vi "Delete.vi"(8 "error in (no error)":errorcluster, 11 "ByRefClass in":refnum<class "ClassByRef.lvclass">) -> (0 "error out":errorcluster, 2 "data value":refnum<class "ClassByRef.lvclass">)   [LabVIEW 2021, in "ClassUtilities.lvlib" / "ClassByRef.lvclass"]
uses:
  ClassByRef.lvclass
  ClassByRef.lvclass/ClassByRef.ctl
  1b75d173-0b49-4d93-ac18-66fa675136c9.vi
  GetExitEvent.vi
  GetRef.vi
  GetExitEvent.vi/d78f5ac1-b881-48f7-a86d-8a9fda2b8e49.vi
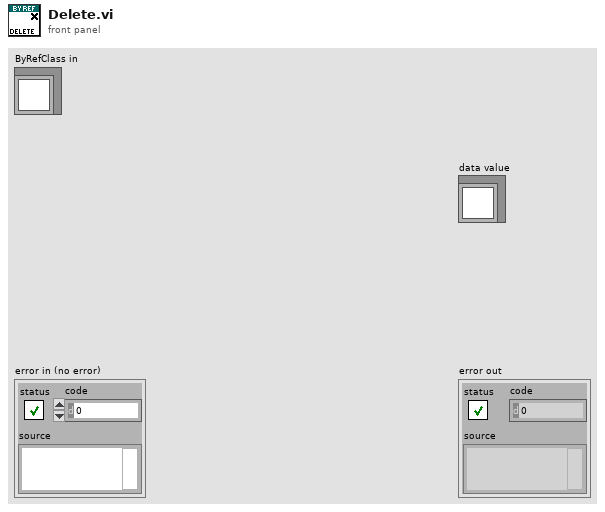
[diagram p1: front panel]
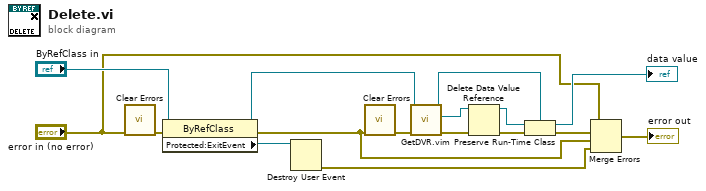
[diagram p0: block diagram]
diagram:
  n1 = call <vilib>:"Clear Errors.vi"("error in (no error)"="error in (no error)") -> ("error out"=w7:errorcluster)  [unwired: 5 in, 1 out]
  n2 = property class="ByRefClass"(reference="ByRefClass in", error in=w7) -> (reference out=w2:refnum<class "ClassByRef.lvclass">, error out=w10:errorcluster, "Protected:ExitEvent"=w8:refnum<user-event>)
  n3 = Destroy User Event(user event=w8) -> (error out=w4:errorcluster)  [unwired: 1 in]
  n4 = call <vilib>:"Clear Errors.vi"("error in (no error)"=w10) -> ("error out"=w3:errorcluster)  [unwired: 5 in, 1 out]
  n5 = call "GetDVR.vim"("error in (no error)"=w3, "ByRefClass in"=w2) -> ("error out"=w16:errorcluster, "DVR"=w15:refnum<data-value>, "ByRefClass out"=w1:refnum<class "ClassByRef.lvclass">)  [unwired: 7 in]
  n6 = Delete Data Value Reference(data value reference=w15, error in=w16) -> (data value=w14:refnum<class "ClassByRef.lvclass">, error out=w12:errorcluster)
  n7 = Preserve Run-Time Class(object in=w14, error in=w12, 2:w1) -> (object out=→"data value":refnum<class "ClassByRef.lvclass">, error out=w11:errorcluster)
  n8 = Merge Errors("error in (no error)", w11, w10, w4) -> (→"error out":errorcluster)
